vi "DG535InstrStatus.vi"(8 "error in":errorcluster, 11 "VISA resource name":refnum<visa-resource-name>) -> (0 "error out":errorcluster, 2 "error found":bool, 3 "duplicate VISA resource":refnum<visa-resource-name>)   [LabVIEW 2012, in "SRS_DG535_Lib.lvlib"]
doc: "This support subVI queries the instrument's error status bits which reports an execution error .\n ERROR FOUND is set to TRUE when an out of range parameter or a delay linkage error causes an execution error . \n This subVI is used in the function subVIs after setting some or all of the instrument's functions .\n The status of ERROR FOUND is then used in the function subVIs to report an error for the parameter that caused it ."
uses:
  SRS_DG535_Lib.lvlib
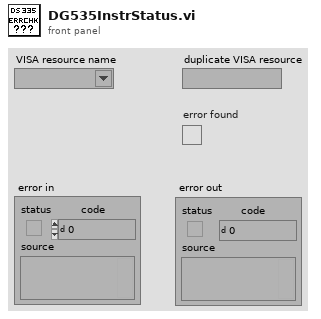
[diagram p1: front panel]
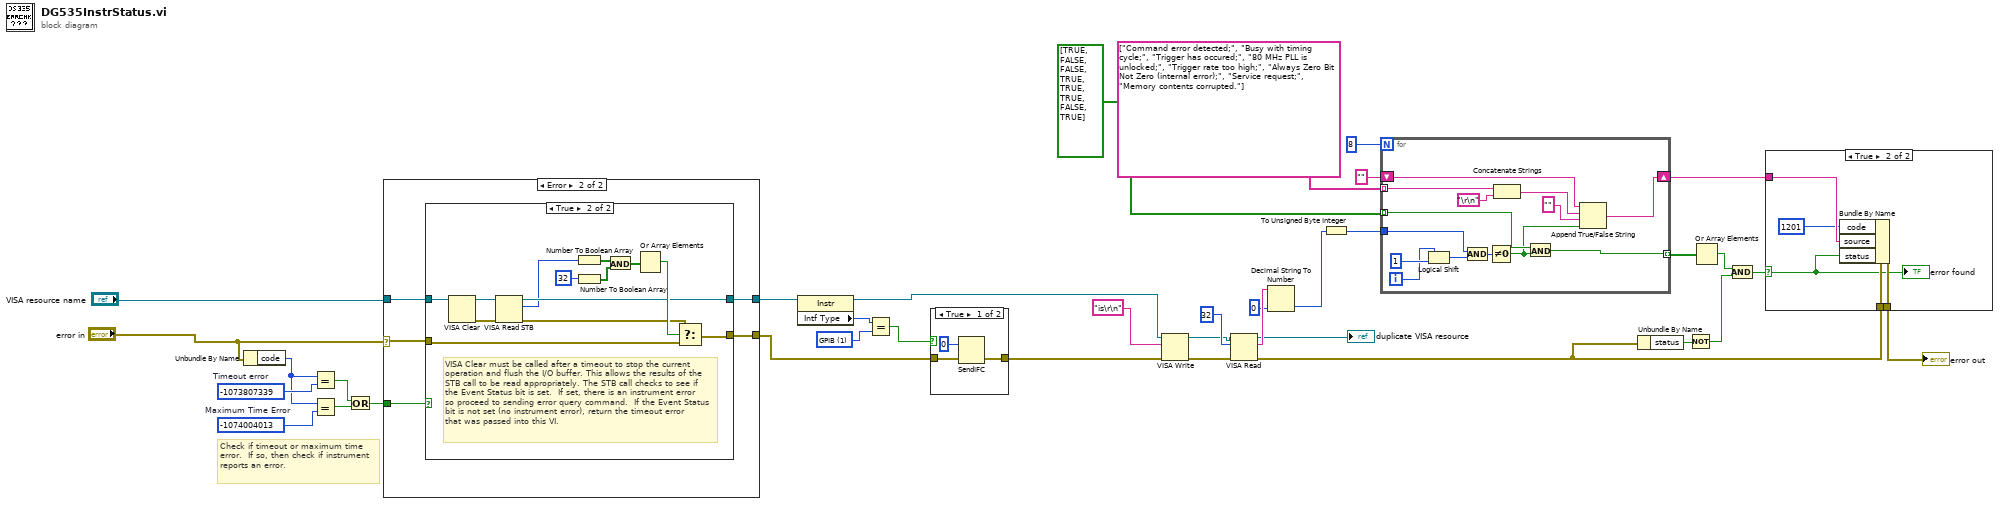
[diagram p0: block diagram]
diagram:
  w11 = -1074004013  # Maximum Time Error
  w13 = -1073807339  # Timeout error
  w16 = u16 1 items=["GPIB"=1, "VXI"=2, "GPIB-VXI"=3, "Serial"=4, "PXI"=5, "TCPIP"=6, "USB"=7, "FireWire"=9] ("Interface Information:Interface Type")
  # "Check if timeout or maximum time error.  If so, then check if instrument reports an error."
  n1 = Unbundle By Name("error in") -> ("code"=w12:i32)
  n2 = Equal?(x=w12, y=w13) -> (x = y?=w9:bool)
  n3 = Equal?(x=w12, y=w11) -> (x = y?=w10:bool)
  n4 = Or(x=w9, y=w10) -> (x .or. y?=w8:bool)
  n5 = case shown="Error" "error in" {
    selector: "error in" -> [w36 w40]
    tunnel: "VISA resource name" -> [w37 w42]
    tunnel: [w37 w41] -> w7
    tunnel: [w36 w39] -> w6
    tunnel: w8 -> [_ w38]
    frame No Error {
    }
    frame Error {
      n6 = case shown="True" w38 {
        tunnel: w42 -> [w44 w50]
        tunnel: [w44 w47] -> w41
        tunnel: w40 -> [w43 w53]
        tunnel: [w43 w52] -> w39
        frame False {
          # "Error code not a timeout, so best to pass on to user."
        }
        frame True {
          # "VISA Clear must be called after a timeout to stop the current operation and flush the I/O buffer. This allows the results of the  STB call to be read appropriately. The STB call checks to see if the Event Status bit is set.  If set, there is an instrument error so proceed to sending error query command.  If the Event Status bit is not set (no instrument error), return the timeout error that was passed into this VI."
          n7 = VISA Clear(VISA resource name=w50) -> (VISA resource name out=w49:refnum<visa-resource-name>, error out=w48:errorcluster)  [unwired: 1 in]
          n8 = VISA Read STB(8:w48, 11:w49) -> (0:w46:errorcluster, 2:w45:u16, 3:w47:refnum<visa-resource-name>)
          n9 = Number To Boolean Array(number=w45) -> (Boolean array=w54:bool[])
          n10 = Number To Boolean Array(number=32) -> (Boolean array=w56:bool[])
          n11 = And(x=w54, y=w56) -> (x .and. y?=w55:bool[])
          n12 = Or Array Elements(Boolean array=w55) -> (logical OR=w51:bool)
          n13 = Select(t=w46, s=w51, f=w53) -> (s? t:f=w52:errorcluster)
        }
      }
    }
  }
  n14 = property class="Instr"(reference=w7) -> (reference out=w4:refnum<visa-resource-name>, "Intf Type"=w15:u16)  [unwired: 1 in, 1 out]
  n15 = Equal?(x=w15, y=w16) -> (x = y?=w14:bool)
  n16 = case shown="True" w14 {
    tunnel: w6 -> [w59 w61]
    tunnel: [w58 w61] -> w2
    frame True {
      n17 = SendIFC(2:w59, 3:0) -> (0:w58:errorcluster)  [unwired: 1 out]
    }
    frame False {
    }
  }
  n18 = VISA Write(VISA resource name=w4, write buffer="is\r\n" ("command string"), error in (no error)=w2) -> (error out=w30:errorcluster)  [unwired: 2 out]
  n19 = VISA Read(VISA resource name=w4, byte count=u32 32, error in (no error)=w30) -> (VISA resource name out=→"duplicate VISA resource":refnum<visa-resource-name>, read buffer=w29:string, error out=w35:errorcluster)  [unwired: 1 out]
  n20 = Decimal String To Number(string=w29, default (0L)=0 ("default (0 I32)")) -> (number=w1:i32)  [unwired: 1 in, 1 out]
  n21 = To Unsigned Byte Integer(number=w1) -> (unsigned 8bit integer=w26:u8)
  n22 = for {
    N: 8 -> [_]
    tunnel: w26 -> [w72]
    shift-right: [w69] -> w20
    shift-left: "" ("output string") -> [w70]
    tunnel: string[] ["Command error detected;", "Busy with timing cycle;", "Trigger has occured;", "80 MHz PLL is unlocked;", "Trigger rate too high;", "Always Zero Bit Not Zero (internal error);", "Service request;", "Memory contents corrupted."] -> [w68] mode=indexing
    tunnel: [w66] -> w23 mode=indexing
    tunnel: bool[] [TRUE, FALSE, FALSE, TRUE, TRUE, TRUE, FALSE, TRUE] -> [w65] mode=indexing
    i -> [w74]
    n23 = Logical Shift(y=w74, x=u8 1 ("y")) -> (x << y=w73:u8)
    n24 = And(x=w72, y=w73) -> (x .and. y?=w71:u8)
    n25 = Not Equal To 0?(x=w71) -> (x != 0?=w64:bool)
    n26 = Concatenate Strings(w68, "\r\n") -> (w63:string)
    n27 = And(x=w65, y=w64) -> (x .and. y?=w66:bool)
    n28 = Append True/False String(1:w64, 2:"" ("false string"), 3:w63, 4:w70) -> (0:w69:string)
  }
  n29 = Unbundle By Name(w35) -> ("status"=w32:bool)
  n30 = Not(x=w32) -> (.not. x?=w31:bool)
  n31 = Or Array Elements(Boolean array=w23) -> (logical OR=w22:bool)
  n32 = And(x=w22, y=w31) -> (x .and. y?=w19:bool)
  n33 = case shown="True" w19 {
    selector: w19 -> [_ w77]
    tunnel: w35 -> [w76 w81]
    tunnel: [w76 w80] -> w21
    tunnel: w20 -> [_ w79]
    frame False {
    }
    frame True {
      n34 = Bundle By Name(cluster=w81, "code"=1201, "source"=w79, "status"=w77) -> (w80:errorcluster)
      "error found" <- w77
    }
  }
  "error out" <- w21
